vi "calcSystemDerivedParameters.vi"(8 "error in (no error)":errorcluster, 11 "ComponentData in":refnum<class "ComponentData.lvclass">) -> (0 "error out":errorcluster, 3 "ComponentData out":refnum<class "ComponentData.lvclass">)   [LabVIEW 2013, in "ComponentData.lvlib" / "ComponentData.lvclass"]
uses:
  <userlib>/Common/Component/common_application/RT/ComponentData/ComponentData/ComponentData.lvclass
  <userlib>/Common/Component/common_application/RT/ComponentData/ComponentData/ComponentData.lvclass/ComponentData.ctl
  <userlib>/Common/Component/common_application/RT/ComponentData/LoopTimer/LoopTimer.lvclass
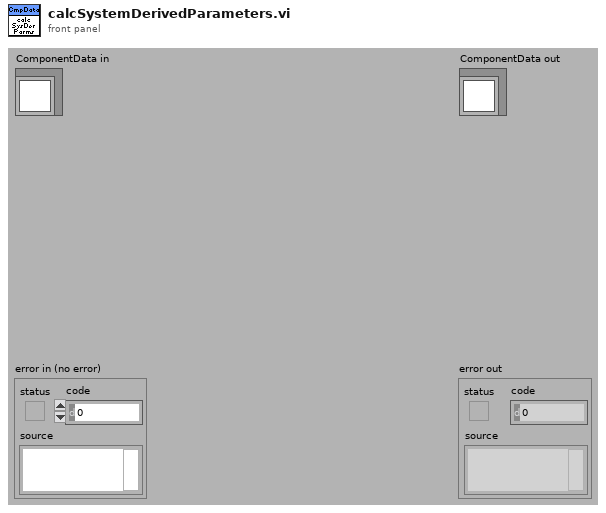
[diagram p1: front panel]
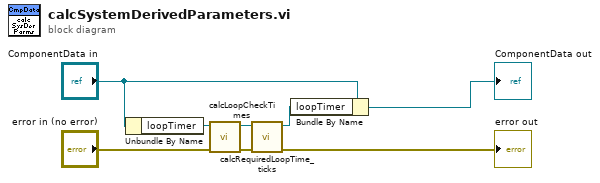
[diagram p0: block diagram]
diagram:
  n1 = Unbundle By Name("ComponentData in") -> ("loopTimer"=w4:refnum<class "LoopTimer.lvclass">)
  n2 = call <userlib>:"calcLoopCheckTimes.vi"("error in (no error)"="error in (no error)", "LoopTimer in"=w4) -> ("error out"=w3:errorcluster, "LoopTimer out"=w2:refnum<class "LoopTimer.lvclass">)  [unwired: 8 in]
  n3 = call <userlib>:"calcRequiredLoopTime_ticks.vi"("error in (no error)"=w3, "LoopTimer in"=w2) -> ("error out"=→"error out":errorcluster, "LoopTimer out"=w1:refnum<class "LoopTimer.lvclass">)  [unwired: 8 in]
  n4 = Bundle By Name(cluster="ComponentData in", "loopTimer"=w1) -> (→"ComponentData out":refnum<class "ComponentData.lvclass">)
